vi "M14_Intake_Hardware_Globals.vi"() -> ()   [LabVIEW 2019]
panel:
  in  "Intake_Pnuematic_Mode":enum16{"Expanded", "Retracted"}(ring)
  in  "Intake Pnuematic":string="Intake Pnuematic"
  in  "Intake Motor A":string="Intake Motor A"
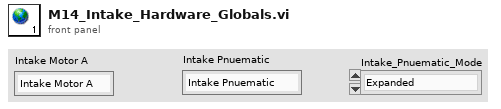
[diagram p1: front panel]
diagram:
